vi "HEATdll.vi"(8 "error in (no error)":errorcluster, 11 "Inputs":cluster{"t":dbl, "D":dbl, "z":dbl[]}) -> (0 "error out":errorcluster, 3 "Outputs":T1)   [LabVIEW 2016]
doc: "subroutine HEATdll(t, d, z, hg, hn, ierr, herr, herr_length)\n\nCompute the ideal-gas gross and net heating values.\n\nINPUTS:\nt -- Temperature [K]\nd -- Molar density [mol/L]\nz -- Composition (array of mole fractions)\n\nOUTPUTS:\nhg -- Gross (or superior) heating value [J/mol]\nhn -- Net (or inferior) heating value [J/mol]\nierr -- Error flag: 0 - Successful 662 - Not all heating values available 665 - Error in chemical formula\nherr -- Error string (character*255)\nherr_length -- length of variable herr (default: 255)"
uses:
  REFPROP.DLL
panel:
  # "REFPROP-HEATdll.vi"
  # "void  HEATdll(double *t, double *D, double *z, double *hg, double *hn, int32_t *ierr, CStr herr, int32_t herr_length)"
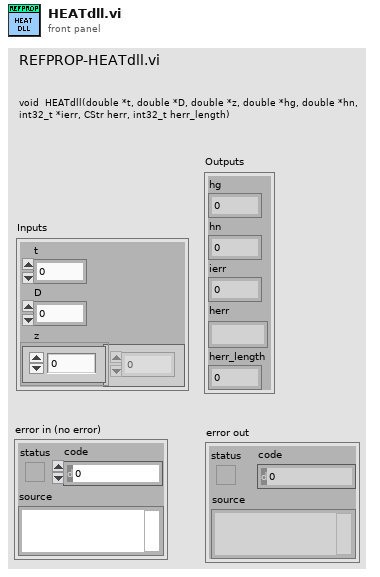
[diagram p1: front panel]
types:
  T1 = cluster{"hg":dbl, "hn":dbl, "ierr":i32, "herr":string, "herr_length":i32}
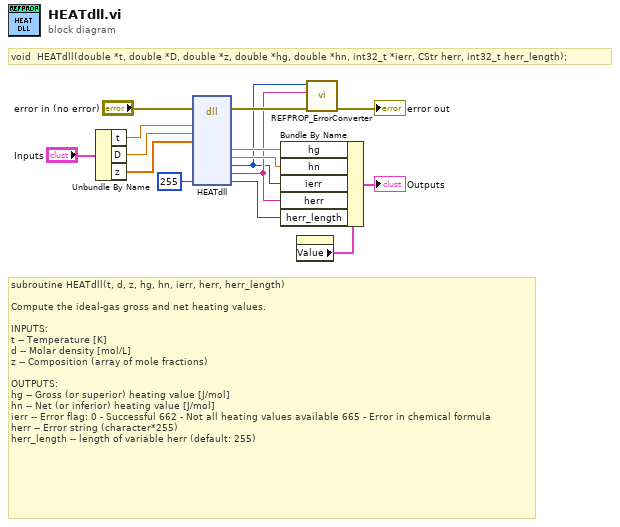
[diagram p0: block diagram]
diagram:
  # "void  HEATdll(double *t, double *D, double *z, double *hg, double *hn, int32_t *ierr, CStr herr, int32_t herr_length);"
  # "subroutine HEATdll(t, d, z, hg, hn, ierr, herr, herr_length)\n\nCompute the ideal-gas gross and net heating values.\n\nINPUTS:\nt -- Temperature [K]\nd -- Molar density [mol/L]\nz -- Composition (array of mole fractions)\n\nOUTPUTS:\nhg -- Gross (or superior) heating value [J/mol]\nhn -- Net (or inferior) heating value [J/mol]\nierr -- Error flag: 0 - Successful 662 - Not all heating values available 665 - Error in chemical formula\nherr -- Error string (character*255)\nherr_length -- length of variable herr (default: 255)"
  n1 = Unbundle By Name("Inputs") -> ("t"=w10:dbl, "D"=w9:dbl, "z"=w8:dbl[])
  n2 = dll-call lib="S:/009 - Testing/02 - Performance Testing/REFPROP/REFPROP.*" fn="HEATdll"(error in="error in (no error)", "t"=w10, "D"=w9, "z"=w8, "herr_length"=255 ("ln")) -> (error out=w14:errorcluster, "hg"=w3:dbl, "hn"=w4:dbl, "ierr"=w1:i32, "herr"=w2:string, "herr_length"=w5:i32)  [unwired: 10 in, 1 out]
  n3 = property on="Outputs" class="Clust (strict)"() -> ("Value"=w7:T1)  [unwired: 2 in, 2 out]
  n4 = Bundle By Name(cluster=w7, "hg"=w3, "hn"=w4, "ierr"=w1, "herr"=w2, "herr_length"=w5) -> (→"Outputs":T1)
  n5 = call "REFPROP_ErrorConverter.vi"("error in (no error)"=w14, "Error Message"=w2, "Error Code"=w1) -> ("error out"=→"error out":errorcluster)  [unwired: 8 in]
